vi "1-1.vi"() -> ()   [LabVIEW 2019, in "AoC2022.lvlib"]
uses:
  AoC2022.lvlib
panel:
  out "result":i32
  out "max value":i32
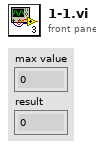
[diagram p1: front panel]
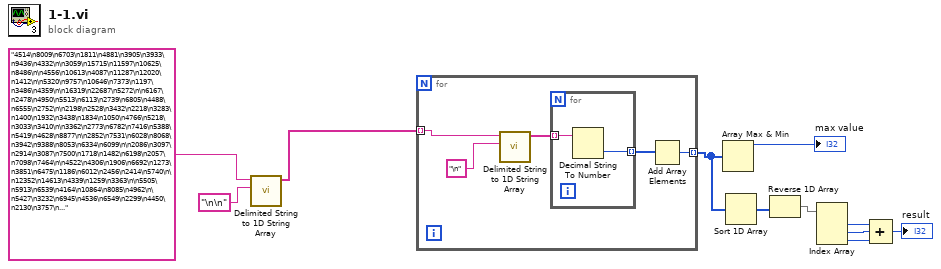
[diagram p0: block diagram]
diagram:
  n1 = call <vilib>:"Delimited String to 1D String Array.vi"("delimiter"="\n\n", "delimited string"="4514\n8009\n6703\n1811\n4881\n3905\n3933\n9436\n4332\n\n3059\n15715\n11597\n10625\n8486\n\n4556\n10613\n4087\n11287\n12020\n1412\n\n5320\n9757\n10646\n7373\n1197\n3486\n4359\n\n16319\n22687\n5272\n\n6167\n2478\n4950\n5513\n6113\n2739\n6805\n4488\n6555\n2752\n\n2198\n2528\n3432\n2218\n3283\n1400\n1932\n3438\n1834\n1050\n4766\n5218\n3033\n3410\n\n3362\n2773\n6782\n7416\n5388\n5419\n4628\n8877\n\n2852\n7531\n6028\n8068\n3942\n9388\n8053\n6334\n6099\n\n2086\n3097\n2914\n3087\n7500\n1718\n1482\n6198\n2057\n7098\n7464\n\n4522\n4306\n1906\n6692\n1273\n3851\n6475\n1186\n6012\n2456\n2414\n5740\n\n12352\n14613\n4339\n1259\n3363\n\n5505\n5913\n6539\n4164\n10864\n8085\n4962\n\n5427\n3232\n6945\n4536\n6549\n2299\n4450\n2130\n3757\n...") -> ("string array"=w9:string[])  [unwired: 9 in]
  n2 = for {
    tunnel: w9 -> [w15] mode=indexing
    tunnel: [w12] -> w7 mode=indexing
    n3 = call <vilib>:"Delimited String to 1D String Array.vi"("delimiter"="\n", "delimited string"=w15) -> ("string array"=w14:string[])  [unwired: 9 in]
    n4 = for {
      tunnel: w14 -> [w18] mode=indexing
      tunnel: [w17] -> w13 mode=indexing
      n5 = Decimal String To Number(string=w18) -> (number=w17:i32)  [unwired: 2 in, 1 out]
    }
    n6 = Add Array Elements(numeric array=w13) -> (sum=w12:i32)
  }
  n7 = Array Max & Min(array=w7) -> (max value=→"max value":i32)  [unwired: 3 out]
  n8 = Sort 1D Array(array=w7) -> (sorted array=w6:i32[])
  n9 = Reverse 1D Array(array=w6) -> (reversed array=w5:i32[])
  n10 = Index Array(array=w5) -> (element #1=w4:i32, element #2=w3:i32, element #3=w2:i32)  [unwired: 3 in]
  n11 = Compound Arithmetic op=ADD(w4, w3, w2) -> (→"result":i32)
